vi "TimeInData.vi"(6 "clSampleDataArray":T1, 9 "SensorTime":timestamp, 10 "AnalysisCycles":dbl, 11 "F0":u32) -> (1 "AnalysisFirst":bool, 2 "NoDataInWindow":bool)   [LabVIEW 2018, in "AnalysisPlugins.lvlib" / "FitterBase.lvclass"]
uses:
  FitterBase.lvclass
  AnalysisPluginBaseClass/Typedefs/SampleDataInput.ctl
  AnalysisPluginBaseClass/AnalysisPluginsBase.lvclass
panel:
  out "DataTime":timestamp
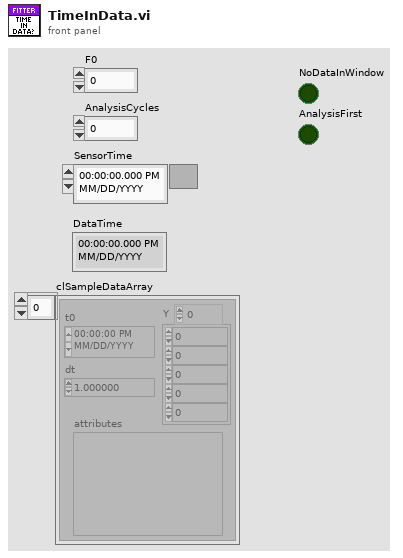
[diagram p1: front panel]
types:
  T1 = typedef "AnalysisPlugins.lvlib/AnalysisPluginsBase.lvclass/SampleDataInput.ctl" = waveform(dbl)[]
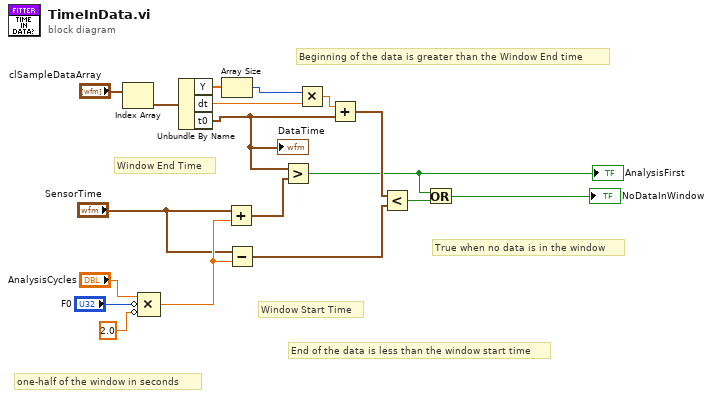
[diagram p0: block diagram]
diagram:
  # "True when no data is in the window"
  # "End of the data is less than the window start time"
  # "Window Start Time"
  # "Window End Time"
  # "one-half of the window in seconds"
  # "Beginning of the data is greater than the Window End time"
  n1 = Index Array(array="clSampleDataArray") -> (element=w17:waveform(dbl))  [unwired: 1 in]
  n2 = Compound Arithmetic op=MULTIPLY("AnalysisCycles", invert "F0", invert 2.0 ("value")) -> (w8:dbl)
  n3 = Unbundle By Name(w17) -> ("Y"=w16:dbl[], "dt"=w14:dbl, "t0"=w1:timestamp)
  "DataTime" <- w1
  n4 = Array Size(array=w16) -> (size(s)=w15:i32)
  n5 = Add(x="SensorTime", y=w8) -> (x+y=w6:timestamp)
  n6 = Subtract(x="SensorTime", y=w8) -> (x-y=w5:timestamp)
  n7 = Greater?(x=w1, y=w6) -> (0:w2:bool)
  "AnalysisFirst" <- w2
  n8 = Multiply(x=w15, y=w14) -> (x*y=w13:dbl)
  n9 = Add(x=w13, y=w1) -> (x+y=w12:timestamp)
  n10 = Less?(x=w12, y=w5) -> (x < y?=w4:bool)
  n11 = Or(x=w2, y=w4) -> (x .or. y?=→"NoDataInWindow":bool)
